vi "Read Control Refnum Values and Set Object Items.vi"(5 "enable LabVIEW extensions? (T)":bool=TRUE, 7 "$Path or Item Name":string caption="Object $Path or Item Name", 8 "error in (no error)":errorcluster, 9 "Control References":refnum<vi>[](array[refnum]), 10 "Object Offset":i32, 11 "JSON":string="{}") -> (0 "error out":errorcluster, 3 "<JSON>":string)   [LabVIEW 2021, in "json.facade.lvlib"]
doc: "Using an Array of Control References, insert (or replace) multiple items into a JSON Object specified by the Object $Path. The item names are the Labels of the Controls, and the item values are the Control Values (converted to JSON).\n\nIf the path specified does not exist, but its immediate parent does, then a new object is created.\n\nSee Detailed Help on JSON Path expressions supported by JSONtext."
uses:
  json.facade.lvlib
  jsontext/LVClass Serializer/JSONtext LVClass Serializer.lvclass
  jsontext/JSONtext.lvlib
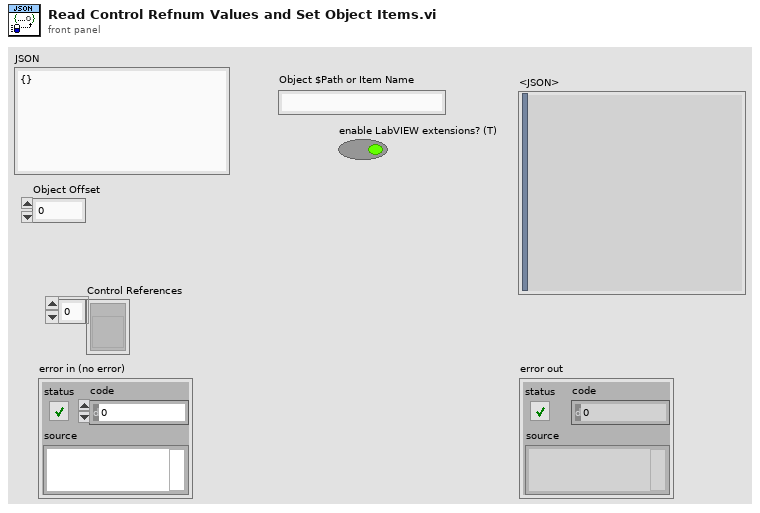
[diagram p1: front panel]
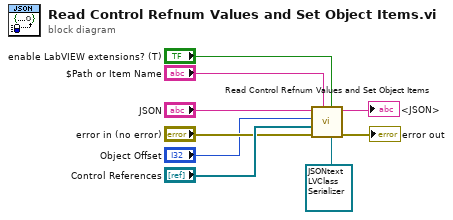
[diagram p0: block diagram]
diagram:
  n1 = call "Read Control Refnum Values and Set Object Items.vi"("LVClass Serializer"=refnum<class "JSONtext LVClass Serializer.lvclass"> refnum, "enable LabVIEW extensions? (T)"="enable LabVIEW extensions? (T)", "$Path or Item Name"="$Path or Item Name", "error in (no error)"="error in (no error)", "Control References"="Control References", "Object Offset"="Object Offset", "JSON"="JSON") -> ("error out"=→"error out":errorcluster, "<JSON>"=→"<JSON>":string)  [unwired: 3 in]
